vi "FindNode.vi"(5 "UID":i32, 9 "VI_AST in":refnum<class "VI_AST.lvclass">) -> (3 "VI_AST out":refnum<class "VI_AST.lvclass">, 4 "index":i32)   [LabVIEW 2014, in "VI_AST.lvclass"]
uses:
  VI_AST.lvclass
  VI_AST.lvclass/VI_AST.ctl
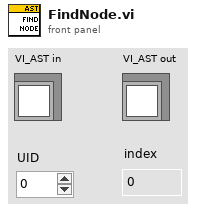
[diagram p1: front panel]
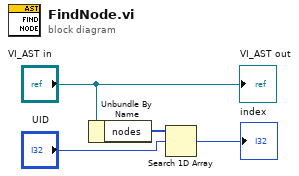
[diagram p0: block diagram]
diagram:
  n1 = Unbundle By Name("VI_AST in") -> ("nodes"=w2:i32[])
  n2 = Search 1D Array(1D array=w2, element="UID") -> (index of element=→"index":i32)  [unwired: 1 in]
  "VI_AST out" <- "VI_AST in"
